vi "Check Stopping.vi"(10 "Unified Actor Lifetime":T1) -> (2 "Stopping":bool)   [LabVIEW 2020, in "jettl.lvlib"]
uses:
  jettl.lvlib
  Unified Actor Lifetime.ctl
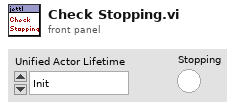
[diagram p1: front panel]
types:
  T1 = typedef "jettl.lvlib/Unified Actor Lifetime.ctl" = enum16{"Init", "Spawn", "Setup", "Teardown Before Running", "Running", "Stop Called", "Stopping With Children", "Stopping Without Children", "Teardown After Running", "Stopped"}
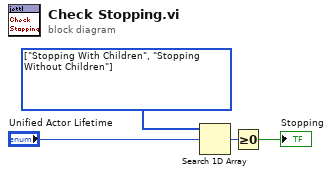
[diagram p0: block diagram]
diagram:
  w3 = T1[] [enum."Stopping With Children", enum."Stopping Without Children"] items=["Init", "Spawn", "Setup", "Teardown Before Running", "Running", "Stop Called", "Stopping With Children", "Stopping Without Children", "Teardown After Running", "Stopped"]
  n1 = Search 1D Array(1D array=w3, element="Unified Actor Lifetime") -> (index of element=w4:i32)  [unwired: 1 in]
  n2 = Greater Or Equal To 0?(x=w4) -> (x >= 0?=→"Stopping":bool)
